vi "ServerRunProcess.vi"(2 "Process Name":string, 3 "Process Reference in":refnum<vi>, 9 "Error in (no error)":errorcluster) -> (0 "Process Reference out":refnum<vi>, 6 "Error out":errorcluster)   [LabVIEW 2009]
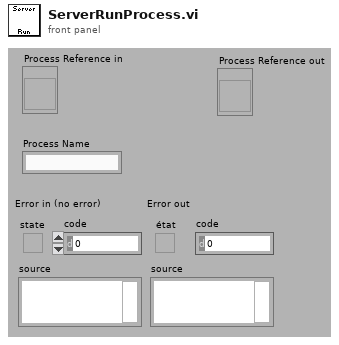
[diagram p1: front panel]
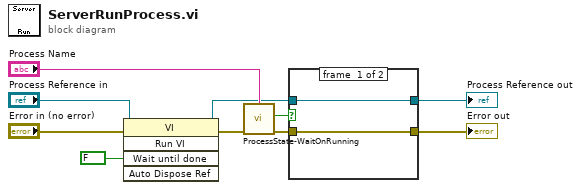
[diagram p0: block diagram]
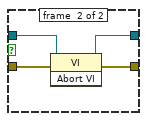
[diagram p2: hidden frame]
diagram:
  n1 = invoke class="VI" method="Run VI"(reference="Process Reference in", error in="Error in (no error)", "Wait until done"=FALSE ("Attente synchrone")) -> (reference out=w5:refnum<vi>, error out=w8:errorcluster)  [unwired: 2 in, 3 out]
  n2 = call "ProcessState-WaitOnRunning.vi"("PROCESS"="Process Name", "error in (no error)"=w8) -> ("timed out?"=w1:bool, "error out"=w4:errorcluster)  [unwired: 6 out]
  n3 = case shown="True" w1 {
    tunnel: w5 -> [w11 w16]
    tunnel: w4 -> [w12 w15]
    tunnel: [w12 w14] -> w3
    tunnel: [w11 w13] -> w2
    frame #0 {
    }
    frame #1 {
      n4 = invoke class="VI" method="Abort VI"(reference=w16, error in=w15) -> (reference out=w13:refnum<vi>, error out=w14:errorcluster)  [unwired: 1 in, 1 out]
    }
  }
  "Process Reference out" <- w2
  "Error out" <- w3
